vi "TCP - Read MAC Address and Serial Number.vi"(8 "error in":errorcluster, 11 "IP Address":string) -> (0 "error out":errorcluster, 3 "DAQiFi Device - Basic Properties":T1)   [LabVIEW 2020]
uses:
  TypeDefs/TypeDef - Cluster of DAQiFi Device Properties.ctl
  TypeDefs/Enum - Connection Type.ctl
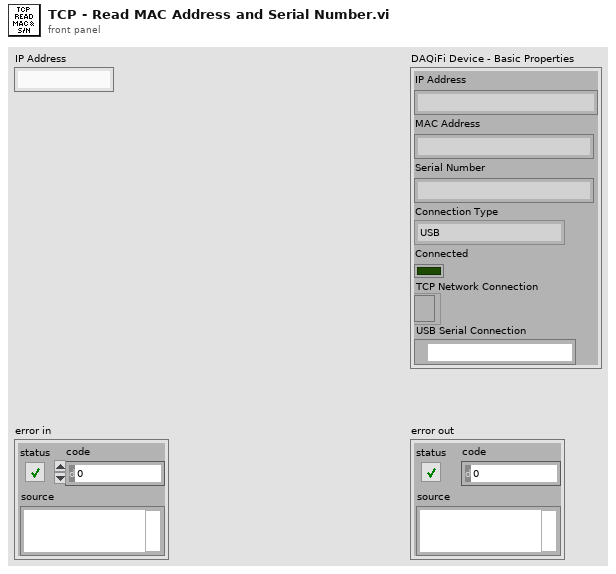
[diagram p1: front panel]
types:
  T1 = typedef "TypeDef - Cluster of DAQiFi Device Properties.ctl" = cluster{"IP Address":string, "MAC Address":string, "Serial Number":string, "Connection Type":T2, "Connected":bool, "TCP Network Connection":refnum<k5>, "USB Serial Connection":refnum<visa-resource-name>}
  T2 = typedef "Enum - Connection Type.ctl" = enum16{"USB", "TCP"}
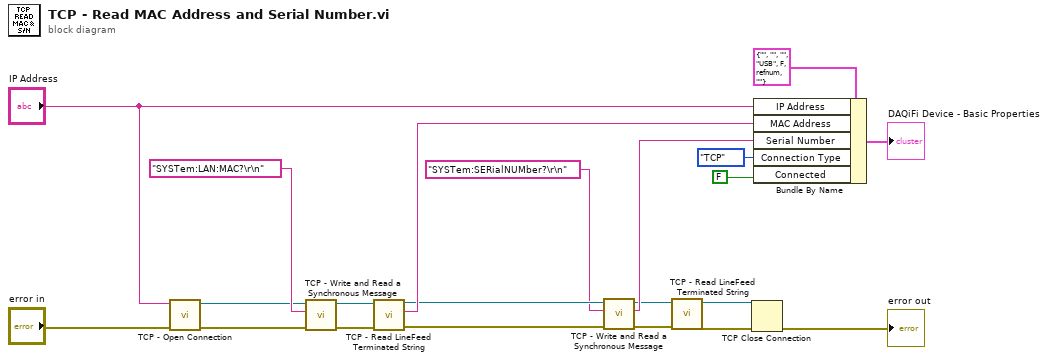
[diagram p0: block diagram]
diagram:
  n1 = call "TCP - Open Connection.vi"("error in (no error)"="error in", "DAQ IP Address"="IP Address") -> ("error out"=w2:errorcluster, "TCP Network Connection out"=w3:refnum<k5>)  [unwired: 8 in]
  n2 = call "TCP - Write and Read a Synchronous Message.vi"("error in"=w2, "Message to Send"="SYSTem:LAN:MAC?\r\n", "TCP Network Connection in"=w3) -> ("error out"=w6:errorcluster, "TCP Network Connection out"=w5:refnum<k5>)  [unwired: 6 in, 1 out]
  n3 = call "TCP - Read LineFeed Terminated String.vi"("error in"=w6, "TCP Network Connection in"=w5) -> ("error out"=w11:errorcluster, "Received Text"=w16:string, "TCP Network Connection out"=w10:refnum<k5>)  [unwired: 7 in]
  n4 = call "TCP - Write and Read a Synchronous Message.vi"("error in"=w11, "Message to Send"="SYSTem:SERialNUMber?\r\n", "TCP Network Connection in"=w10) -> ("error out"=w9:errorcluster, "Received Text"=w17:string, "TCP Network Connection out"=w8:refnum<k5>)  [unwired: 6 in]
  n5 = call "TCP - Read LineFeed Terminated String.vi"("error in"=w9, "TCP Network Connection in"=w8) -> ("error out"=w12:errorcluster, "TCP Network Connection out"=w13:refnum<k5>)  [unwired: 7 in, 1 out]
  n6 = TCP Close Connection(connection ID=w13, error in (no error)=w12) -> (error out=→"error out":errorcluster)  [unwired: 1 in, 1 out]
  n7 = Bundle By Name(cluster=T1 {"IP Address"="", "MAC Address"="", "Serial Number"="", "Connection Type"=enum."USB", "Connected"=FALSE, "TCP Network Connection"=refnum, "USB Serial Connection"=""} ("DAQiFi Device - Basic Properties"), "IP Address"="IP Address", "MAC Address"=w16, "Serial Number"=w17, "Connection Type"=Enum_-_Connection_Type."TCP", "Connected"=FALSE) -> (→"DAQiFi Device - Basic Properties":T1)
